vi "Load Glyph.vi"(8 "error in (no error)":errorcluster, 10 "glyph_index":u32, 11 "face in":i64) -> (0 "error out":errorcluster, 3 "face out":i64)   [LabVIEW 2023, in "Freetype Drawer.lvlib"]
uses:
  Freetype Drawer.lvlib
  libfreetype.dll
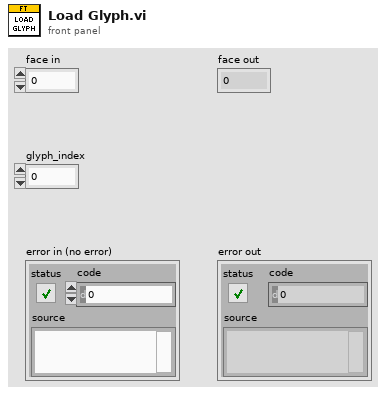
[diagram p1: front panel]
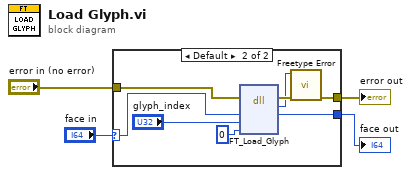
[diagram p0: block diagram]
diagram:
  n1 = case shown="Default" "face in" {
    selector: "face in" -> [w5 w13]
    tunnel: "error in (no error)" -> [w6 w14]
    tunnel: [w5 w12] -> w2
    tunnel: [w6 w7] -> w1
    frame 0 {
    }
    frame Default {
      n2 = dll-call lib="E:/Labview/LV 2023/Libs/LV Symbol/Freetype Drawer/Wrappers/libfreetype.dll" fn="FT_Load_Glyph"(error in=w14, "face"=w13, "glyph_index"="glyph_index", "load_flags"=0) -> (error out=w9:errorcluster, "error"=w8:i32, "face"=w12:i64)  [unwired: 4 in, 1 out]
      n3 = call "Freetype Error.vi"("error in (no error)"=w9, "Error"=w8) -> ("error out"=w7:errorcluster)  [unwired: 9 in]
    }
  }
  "error out" <- w1
  "face out" <- w2
